vi "data_ac.vi"() -> ()   [LabVIEW 2026]
uses:
  Control 1.ctl
  <vilib>/DAQmx/read.llb/DAQmx Read (Analog 1D Wfm NChan NSamp).vi
  <vilib>/DAQmx/miscellaneous.llb/DAQmx Fill In Error Info.vi
panel:
  out "data 2":waveform(dbl)[](graph) caption="data"
  in  "stop 2":bool caption="stop"
  out "data":T1
  in  "stop":bool
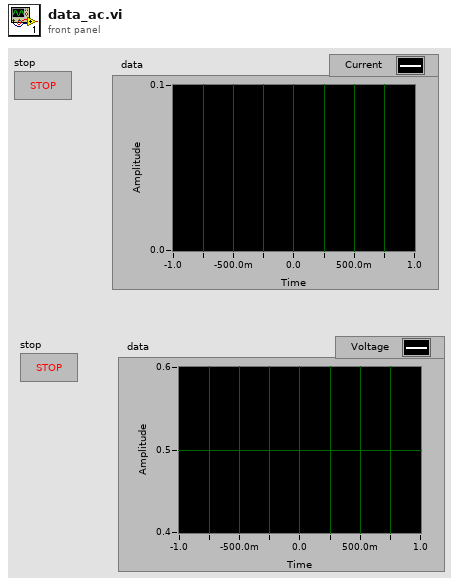
[diagram p1: front panel]
types:
  T1 = typedef "Control 1.ctl" = waveform(dbl)[]
  T2 = enum16{"open", "replace", "create", "open or create", "replace or create", "replace or create with confirmation"}
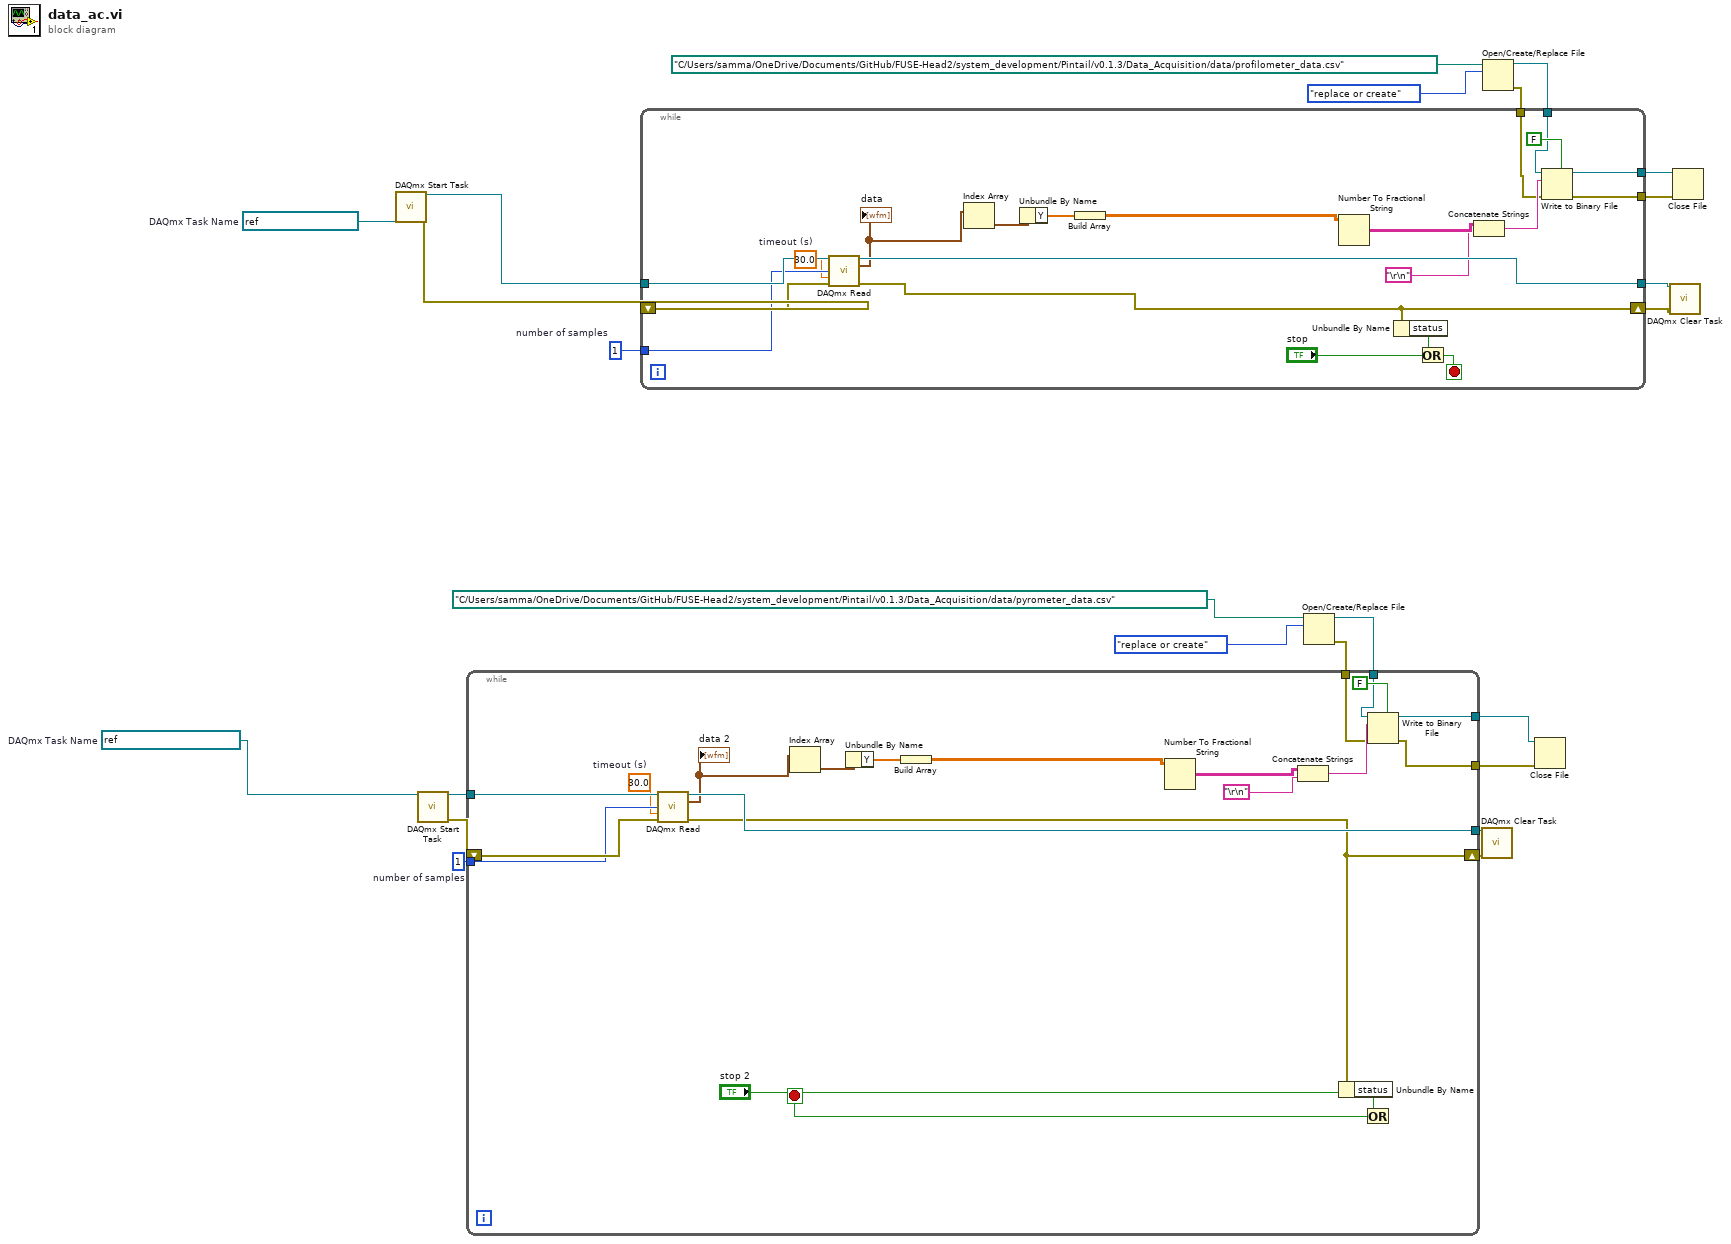
[diagram p0: block diagram]
diagram:
  w17 = 1  # number of samples
  w14 = refnum<k21> "thermoMETER Signal"  # DAQmx Task Name
  w13 = 1  # number of samples
  w20 = refnum<k21> "optoNCDTsignal"  # DAQmx Task Name
  n1 = call <vilib>:"DAQmx Start Task.vi"("task/channels in"=w20) -> ("task out"=w24:refnum<k21>, "error out"=w23:errorcluster)  [unwired: 13 in]
  n2 = call <vilib>:"DAQmx Start Task.vi"("task/channels in"=w14) -> ("task out"=w19:refnum<k21>, "error out"=w18:errorcluster)  [unwired: 13 in]
  n3 = Open/Create/Replace File(file path (use dialog)=path "C:/Users/samma/OneDrive/Documents/GitHub/FUSE-Head2/system_development/Pintail/v0.1.3/Data_Acquisition/data/pyrometer_data.csv", operation (0:open)=T2."replace or create") -> (refnum out=w5:refnum<file>, error out=w6:errorcluster)  [unwired: 4 in, 1 out]
  n4 = while {
    tunnel: w19 -> [w45]
    tunnel: w17 -> [w42]
    tunnel: [w43] -> w15
    shift-right: [w40] -> w16
    shift-left: w18 -> [w44]
    tunnel: w6 -> [w28]
    tunnel: w5 -> [w27]
    tunnel: [w26] -> w2
    tunnel: [w25] -> w1
    stop <- w39 stop-if-true
    w37 = 30.0  # timeout (s)
    n5 = call-poly <vilib>:"DAQmx Read.vi"("task/channels in"=w45, "number of samples per channel"=w42, "timeout"=w37, "error in"=w44) -> ("task out"=w43:refnum<k21>, "data"=w29:waveform(dbl)[], "error out"=w40:errorcluster)  [unwired: 9 in]
    "data 2" <- w29
    n6 = Index Array(array=w29) -> (element=w32:waveform(dbl))  [unwired: 1 in]
    n7 = Unbundle By Name(w32) -> ("Y"=w31:dbl[])
    n8 = Build Array(w31) -> (w30:dbl[][])
    n9 = Number To Fractional String(number=w30) -> (F-format string=w34:string[][])  [unwired: 3 in]
    n10 = Concatenate Strings(w34, "\r\n") -> (w36:string)
    n11 = Unbundle By Name(w40) -> ("status"=w41:bool)
    n12 = Or(x=w41, y="stop 2") -> (x .or. y?=w39:bool)
    n13 = Write to Binary File(file (use dialog)=w27, data=w36, error in=w28, 5:FALSE ("prepend array or string size? (T)")) -> (refnum out=w25:refnum<file>, error out=w26:errorcluster)  [unwired: 2 in, 1 out]
  }
  n14 = call <vilib>:"DAQmx Clear Task.vi"("task in"=w15, "error in"=w16) -> ()  [unwired: 13 in, 1 out]
  n15 = Open/Create/Replace File(file path (use dialog)=path "C:/Users/samma/OneDrive/Documents/GitHub/FUSE-Head2/system_development/Pintail/v0.1.3/Data_Acquisition/data/profilometer_data.csv", operation (0:open)=T2."replace or create") -> (refnum out=w10:refnum<file>, error out=w11:errorcluster)  [unwired: 4 in, 1 out]
  n16 = while {
    tunnel: w24 -> [w66]
    tunnel: w13 -> [w63]
    tunnel: [w64] -> w21
    shift-right: [w61] -> w22
    shift-left: w23 -> [w65]
    tunnel: w11 -> [w50]
    tunnel: w10 -> [w49]
    tunnel: [w48] -> w8
    tunnel: [w47] -> w7
    stop <- w60 stop-if-true
    w58 = 30.0  # timeout (s)
    n17 = call-poly <vilib>:"DAQmx Read.vi"("task/channels in"=w66, "number of samples per channel"=w63, "timeout"=w58, "error in"=w65) -> ("task out"=w64:refnum<k21>, "data"=w56:waveform(dbl)[], "error out"=w61:errorcluster)  [unwired: 9 in]
    "data" <- w56
    n18 = Index Array(array=w56) -> (element=w55:waveform(dbl))  [unwired: 1 in]
    n19 = Unbundle By Name(w55) -> ("Y"=w54:dbl[])
    n20 = Build Array(w54) -> (w53:dbl[][])
    n21 = Number To Fractional String(number=w53) -> (F-format string=w52:string[][])  [unwired: 3 in]
    n22 = Unbundle By Name(w61) -> ("status"=w62:bool)
    n23 = Or(x=w62, y="stop") -> (x .or. y?=w60:bool)
    n24 = Concatenate Strings(w52, "\r\n") -> (w51:string)
    n25 = Write to Binary File(file (use dialog)=w49, data=w51, error in=w50, 5:FALSE ("prepend array or string size? (T)")) -> (refnum out=w47:refnum<file>, error out=w48:errorcluster)  [unwired: 2 in, 1 out]
  }
  n26 = Close File(refnum=w1, error in=w2) -> ()  [unwired: 2 out]
  n27 = call <vilib>:"DAQmx Clear Task.vi"("task in"=w21, "error in"=w22) -> ()  [unwired: 13 in, 1 out]
  n28 = Close File(refnum=w7, error in=w8) -> ()  [unwired: 2 out]
